vi "Read Block Measurements.vi"(7 "Read entire buffer (False)":bool, 8 "error in (no error)":errorcluster, 9 "Timeout (30 secs)":i32=30, 10 "Number of readings (10)":i32=10, 11 "VISA resource name":refnum<visa-resource-name>) -> (0 "error out":errorcluster, 2 "Measurements":dbl[](array[numeric]) format="%#_10g", 3 "VISA resource name out":refnum<visa-resource-name>)   [LabVIEW 2011, in "Fluke 8508.lvlib"]
doc: "This VI reads the specified number of readings from the internal buffer store on the instrument. If an ongoing write exists, the VI will wait until completion of the write operation or until the timeout value is reached.\n\nNOTE: If the instrument is initialized or power cycled, all the existing data in the buffer will be deleted.\n\nNOTE: In some measurement modes, the instruments will timeout before the measurement is complete. For instance, a single measurement can take up to two minutes while the devide is in true ohms mode and configured for an 8 1/2 digit reading. If you run into this problem, set the timeout as necessary using the set timeout VI in the VISA palette."
uses:
  Fluke 8508.lvlib
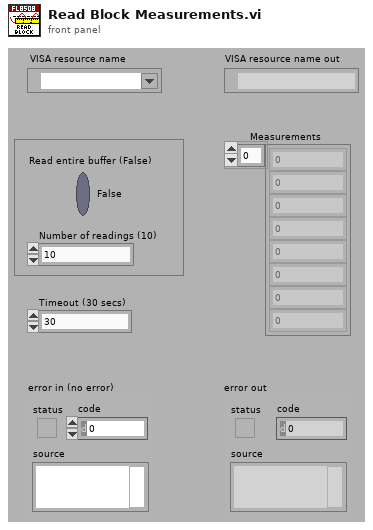
[diagram p1: front panel]
types:
  T1 = cluster{"Status":bool, "Code":i32, "Source (VI Name)":string}
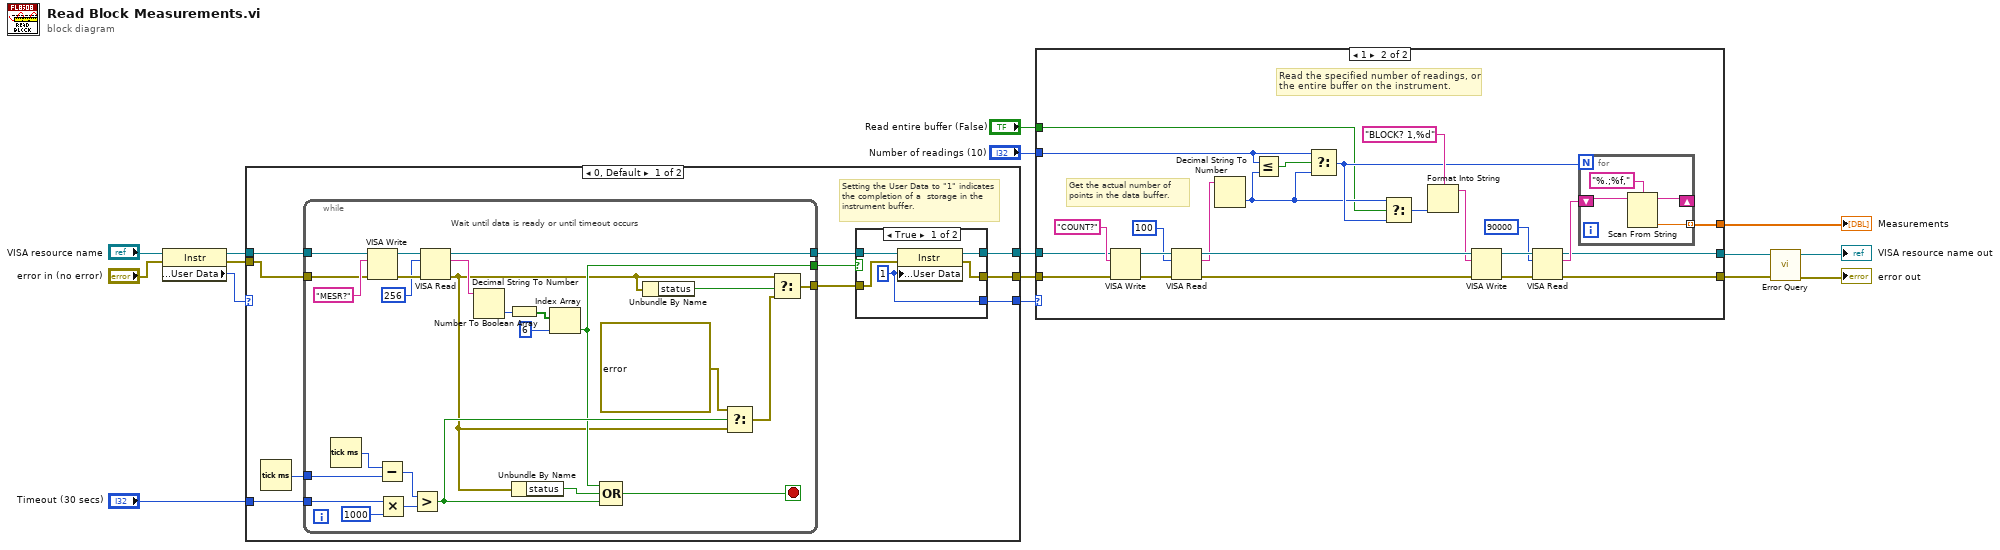
[diagram p0: block diagram]
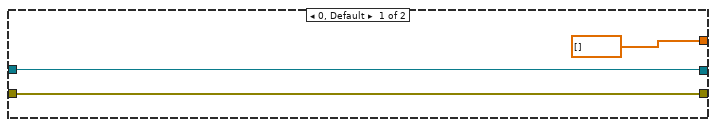
[diagram p2: hidden frame]
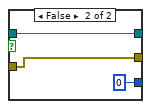
[diagram p3: hidden frame]
diagram:
  n1 = property class="Instr"(reference="VISA resource name", error in="error in (no error)") -> (reference out=w9:refnum<visa-resource-name>, error out=w8:errorcluster, "General Settings:User Data"=w4:u32)
  n2 = case shown="0, Default" w4 {
    selector: w4 -> [_ w61]
    tunnel: w9 -> [w24 w63]
    tunnel: w8 -> [w23 w62]
    tunnel: [w21 w63] -> w7
    tunnel: [w20 w62] -> w6
    tunnel: "Timeout (30 secs)" -> [w25 _]
    tunnel: [w17 w61] -> w3
    frame 0, Default {
      # "Setting the User Data to \"1\" indicates the completion of a  storage in the instrument buffer."
      n3 = Tick Count (ms)() -> (millisecond timer value=w26:u32)
      n4 = while {
        tunnel: w26 -> [w59]
        tunnel: w25 -> [w57]
        tunnel: w24 -> [w47]
        tunnel: w23 -> [w46]
        tunnel: [w39] -> w18
        tunnel: [w38] -> w19
        tunnel: [w37] -> w22
        stop <- w44 stop-if-true
        # "Wait until data is ready or until timeout occurs"
        n5 = Tick Count (ms)() -> (millisecond timer value=w60:u32)
        n6 = VISA Write(VISA resource name=w47, write buffer="MESR?", error in (no error)=w46) -> (VISA resource name out=w45:refnum<visa-resource-name>, error out=w54:errorcluster)  [unwired: 1 out]
        n7 = Subtract(x=w60, y=w59) -> (x-y=w58:u32)
        n8 = Multiply(x=w57, y=u32 1000) -> (x*y=w55:u32)
        n9 = Greater?(x=w58, y=w55) -> (0:w42:bool)
        n10 = VISA Read(VISA resource name=w45, byte count=u32 256, error in (no error)=w54) -> (VISA resource name out=w38:refnum<visa-resource-name>, read buffer=w51:string, error out=w36:errorcluster)  [unwired: 1 out]
        n11 = Decimal String To Number(string=w51) -> (number=w48:i32)  [unwired: 2 in, 1 out]
        n12 = Number To Boolean Array(number=w48) -> (Boolean array=w50:bool[])
        n13 = Unbundle By Name(w36) -> ("status"=w43:bool)
        n14 = Index Array(array=w50, index=6) -> (element=w37:bool)
        n15 = Compound Arithmetic op=OR(w37, w43, w42) -> (w44:bool)
        n16 = Unbundle By Name(w36) -> ("status"=w40:bool)
        n17 = Select(t=T1 {"Status"=TRUE, "Code"=-1073807338, "Source (VI Name)"="<ERR> fl8508a Read Block Measurements\nThe instrument timed out while reading from the internal buffer. This may mean that the instrument is still writing data to the buffer, in which case the timeout value should be increased or that there is no data in the internal buffer. It may also indicate that the instrument is still waiting for the appropriate number of triggers to complete writing data to the buffer i.e. if the external trigger mode is selected and n number of values are to be stored,  the instrument will wait for n triggers before completion."}, s=w42, f=w36) -> (s? t:f=w41:errorcluster)
        n18 = Select(t=w36, s=w40, f=w41) -> (s? t:f=w39:errorcluster)
      }
      n19 = case shown="True" w22 {
        tunnel: [w31 w34] -> w21
        tunnel: [w30 w33] -> w20
        tunnel: w19 -> [w29 w34]
        tunnel: w18 -> [w28 w33]
        tunnel: [w27 u32 0 ("General Settings:User Data")] -> w17
        frame True {
          w27 = u32 1 ("General Settings:User Data")
          n20 = property class="Instr"(reference=w29, error in=w28, "General Settings:User Data"=w27) -> (reference out=w31:refnum<visa-resource-name>, error out=w30:errorcluster)
        }
        frame False {
        }
      }
    }
    frame 1 {
    }
  }
  n21 = case shown="1" w3 {
    tunnel: [dbl[] [] w77] -> w16
    tunnel: [w64 w67] -> w15
    tunnel: [w65 w68] -> w13
    tunnel: w7 -> [w65 w75]
    tunnel: w6 -> [w64 w74]
    tunnel: "Number of readings (10)" -> [_ w69]
    tunnel: "Read entire buffer (False)" -> [_ w70]
    frame 0, Default {
    }
    frame 1 {
      # "Read the specified number of readings, or the entire buffer on the instrument."
      # "Get the actual number of points in the data buffer."
      n22 = VISA Write(VISA resource name=w75, write buffer="COUNT?", error in (no error)=w74) -> (VISA resource name out=w83:refnum<visa-resource-name>, error out=w87:errorcluster)  [unwired: 1 out]
      n23 = VISA Read(VISA resource name=w83, byte count=u32 100, error in (no error)=w87) -> (VISA resource name out=w85:refnum<visa-resource-name>, read buffer=w81:string, error out=w86:errorcluster)  [unwired: 1 out]
      n24 = Decimal String To Number(string=w81) -> (number=w71:i32)  [unwired: 2 in, 1 out]
      n25 = Less Or Equal?(x=w69, y=w71) -> (x <= y?=w80:bool)
      n26 = Select(t=w69, s=w80, f=w71) -> (s? t:f=w73:i32)
      n27 = Select(t=w71, s=w70, f=w73) -> (s? t:f=w72:i32)
      n28 = Format Into String(format string="BLOCK? 1,%d", w72) -> (resulting string=w79:string)  [unwired: 2 in, 1 out]
      n29 = VISA Write(VISA resource name=w85, write buffer=w79, error in (no error)=w86) -> (VISA resource name out=w89:refnum<visa-resource-name>, error out=w90:errorcluster)  [unwired: 1 out]
      n30 = VISA Read(VISA resource name=w89, byte count=u32 90000, error in (no error)=w90) -> (VISA resource name out=w68:refnum<visa-resource-name>, read buffer=w76:string, error out=w67:errorcluster)  [unwired: 1 out]
      n31 = for {
        N: w73 -> [_]
        tunnel: [w93] -> w77 mode=indexing
        shift-right: [w91] -> _
        shift-left: w76 -> [w94]
        n32 = Scan From String(format string="%.;%f,", input string=w94) -> (remaining string=w91:string, output 1=w93:dbl)  [unwired: 3 in, 2 out]
      }
    }
  }
  "Measurements" <- w16
  n33 = call "Error Query.vi"("error in (no error)"=w15, "VISA resource name"=w13) -> ("error out"=→"error out":errorcluster, "VISA resource name out"=→"VISA resource name out":refnum<visa-resource-name>)  [unwired: 6 in, 2 out]
